vi "Eliminate_Zeroes.vi"(10 "Align to First Cases Reported":bool, 11 "Array in":i32[](array[numeric])) -> (3 "Array out":i32[](array[numeric]))   [LabVIEW 2015]
doc: "Eliminates the leading zero elements from the 1D integer array. This can be used to compare two data series that started at different times."
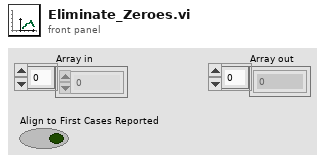
[diagram p1: front panel]
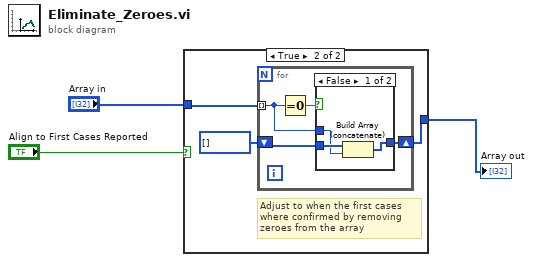
[diagram p0: block diagram]
diagram:
  n1 = case shown="True" "Align to First Cases Reported" {
    tunnel: "Array in" -> [w4 w7]
    tunnel: [w4 w5] -> w2
    frame False {
    }
    frame True {
      # "Adjust to when the first cases\nwhere confirmed by removing\nzeroes from the array"
      n2 = for {
        tunnel: w7 -> [w10] mode=indexing
        shift-right: [w8] -> w5
        shift-left: i32[] [] -> [w9]
        n3 = Equal To 0?(x=w10) -> (x = 0?=w11:bool)
        n4 = case shown="False" w11 {
          tunnel: w10 -> [w12 _]
          tunnel: w9 -> [w14 w15]
          tunnel: [w13 w15] -> w8
          frame False {
            n5 = Build Array (concatenate)(w14, w12) -> (w13:i32[])
          }
          frame True {
          }
        }
      }
    }
  }
  "Array out" <- w2
